vi "MainUI Q.vi"(7 "Enum":enum16{"Initial", "read", "release"}(ring)=enum."read") -> (2 "UI Response Out":refnum<queue>, 3 "UI Receive Out":refnum<queue>)   [LabVIEW 2019]
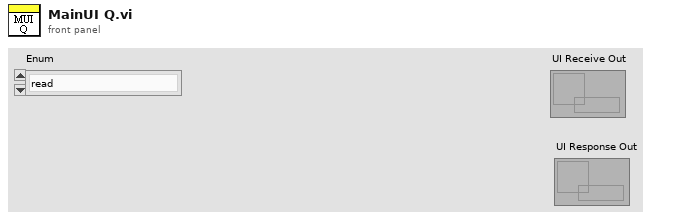
[diagram p1: front panel]
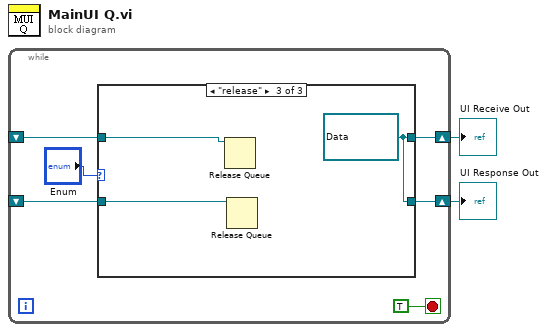
[diagram p0: block diagram]
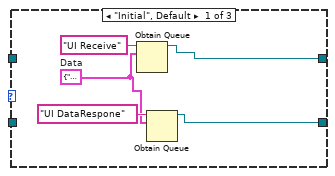
[diagram p2: hidden frame]
diagram:
  n1 = while {
    shift-right: [w6] -> w2
    shift-left: _ -> [w5]
    shift-right: [w4] -> w1
    shift-left: _ -> [w3]
    stop <- TRUE stop-if-true
    n2 = case shown="\"release\"" "Enum" {
      tunnel: [w10 w15 w16] -> w6
      tunnel: w5 -> [_ w15 w18]
      tunnel: [w9 w14 w16] -> w4
      tunnel: w3 -> [_ w14 w17]
      frame "Initial", Default {
        w11 = cluster{"Action":string, "Data":variant} {"Action"="", "Data"=variant}  # Data
        n3 = Obtain Queue(name (unnamed)="UI Receive", element data type=w11) -> (queue out=w10:refnum<queue>)  [unwired: 3 in, 2 out]
        n4 = Obtain Queue(name (unnamed)="UI DataRespone", element data type=w11) -> (queue out=w9:refnum<queue>)  [unwired: 3 in, 2 out]
      }
      frame "read" {
      }
      frame "release" {
        w16 = refnum<queue> refnum ("queue out")
        n5 = Release Queue(queue=w18) -> ()  [unwired: 2 in, 3 out]
        n6 = Release Queue(queue=w17) -> ()  [unwired: 2 in, 3 out]
      }
    }
  }
  "UI Receive Out" <- w2
  "UI Response Out" <- w1
